vi "Update.vi"(8 "error in (no error)":errorcluster caption="entrée d'erreur (pas d'erreur)", 11 "Database Drivers en entrée":refnum<class "Database Drivers.lvclass">) -> (0 "error out":errorcluster caption="sortie d'erreur", 3 "Database Drivers en sortie":refnum<class "Database Drivers.lvclass">)   [LabVIEW 2020, in "Library Instrument & Equipement.lvlib" / "Library Database.lvlib" / "Database Drivers.lvclass"]
uses:
  Database Drivers.lvclass
  <vilib>/addons/database/Command.llb/Cmd Execute.vi
  <vilib>/addons/database/Recordset.llb/Rec Destroy - Command.vi
  <vilib>/addons/database/Command.llb/Cmd Delete.vi
  Database Drivers.lvclass/Database Drivers.ctl
  <vilib>/addons/database/NI_Database_API.lvlib
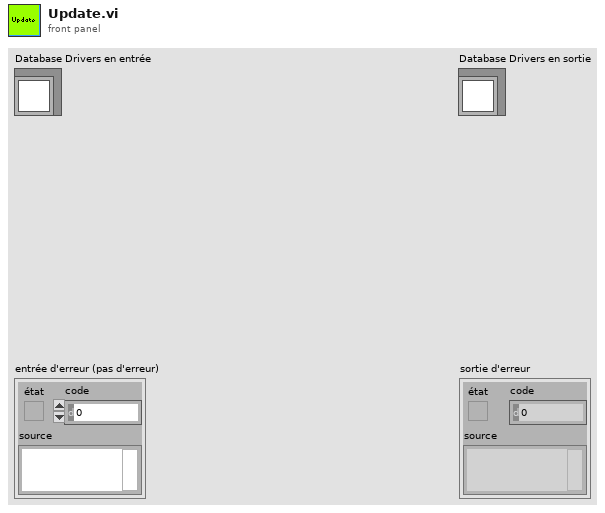
[diagram p1: front panel]
types:
  T1 = typedef "NI_Database_API.lvlib/Conn ObjectReference.ctl" = refnum<k1>
  T2 = typedef "NI_Database_API.lvlib/DB Tools Parameter Info.ctl" = cluster{"parameter name":string, "type":T3, "direction":T4, "value":variant}
  T3 = typedef "NI_Database_API.lvlib/DB Tools DataTypes.ctl" = enum16{"String", "Long (I32)", "Single (SGL)", "Double (DBL)", "Date/Time", "Binary"}
  T4 = typedef "NI_Database_API.lvlib/DB Tools Parameter Dir.ctl" = enum32{"Input", "Output", "Input/Output", "Return Value"}
  T5 = typedef "NI_Database_API.lvlib/Cmd ObjectReference.ctl" = refnum<k1>
  T6 = typedef "NI_Database_API.lvlib/Cmd-Rec Object Reference.ctl" = refnum<k1>
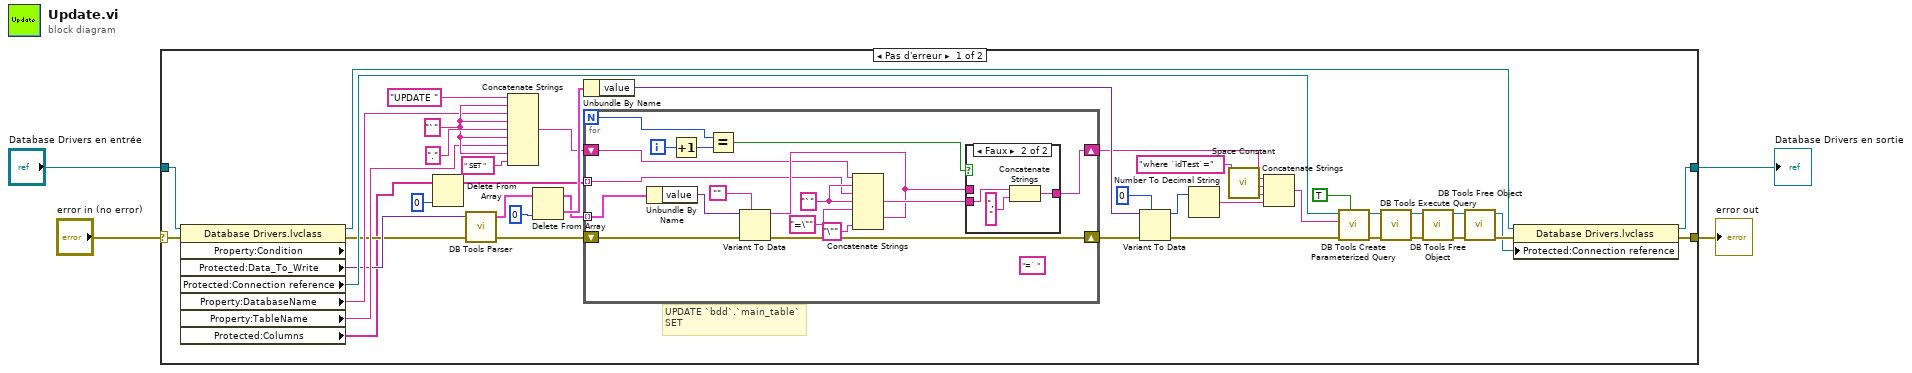
[diagram p0: block diagram]
diagram:
  n1 = case shown="Pas d'erreur" "error in (no error)" {
    selector: "error in (no error)" -> [w45 w69]
    tunnel: [w44 w69] -> w3
    tunnel: [w42 w68] -> w1
    tunnel: "Database Drivers en entrée" -> [w46 w68]
    frame No Error {
      w40 = "`" ("chaîne")
      # "UPDATE `bdd`.`main_table`\nSET"
      n2 = property class="Database Drivers.lvclass" props=["Property:Condition", "Protected:Data_To_Write", "Protected:Connection reference", "Property:DatabaseName", "Property:TableName", "Protected:Columns"](reference=w46, error in=w45) -> (reference out=w43:refnum<class "Database Drivers.lvclass">, error out=w16:errorcluster, "Protected:Data_To_Write"=w21:variant, "Protected:Connection reference"=w23:T1, "Property:DatabaseName"=w39:string, "Property:TableName"=w24:string, "Protected:Columns"=w7:string[])  [unwired: 1 out]
      n3 = Delete From Array(array=w7, index=0 ("indice")) -> (array with subset deleted=w5:string[])  [unwired: 1 in, 1 out]
      n4 = call <vilib>:"DB Tools Parser.vi"("error in (no error)"=w16, "variant"=w21) -> ("error out"=w17:errorcluster, "parameters"=w9:T2[])  [unwired: 2 in]
      n5 = Concatenate Strings("UPDATE " ("chaîne"), w40, w39, w40, "." ("chaîne"), w40, w24, w40, " SET " ("chaîne")) -> (w10:string)
      n6 = Delete From Array(array=w9, index=0 ("indice")) -> (deleted portion=w20:T2, array with subset deleted=w8:T2[])  [unwired: 1 in]
      n7 = Unbundle By Name(w20) -> ("value"=w19:variant)
      n8 = for {
        N -> [w52]
        shift-right: [w60] -> w18
        shift-left: w17 -> [w61]
        shift-right: [w57] -> w15
        shift-left: w10 -> [w56]
        tunnel: w5 -> [w53] mode=indexing
        tunnel: w8 -> [w48] mode=indexing
        i -> [w51]
        w54 = "`" ("chaîne")
        (unwired) "=` "
        n9 = Unbundle By Name(w48) -> ("value"=w63:variant)
        n10 = Increment(x=w51) -> (x+1=w49:i32)
        n11 = Equal?(x=w52, y=w49) -> (x = y?=w50:bool)
        n12 = Variant To Data(error in=w61, type="", Variant=w63) -> (data=w58:string, error out=w60:errorcluster)
        n13 = Concatenate Strings(w56, w54, w53, w54, "=\"", w58, "\"" ("chaîne")) -> (w59:string)
        n14 = case shown="Faux" w50 {
          tunnel: w59 -> [w64 w66]
          tunnel: [w64 w65] -> w57
          tunnel: w58 -> [_ _]
          frame True {
          }
          frame False {
            n15 = Concatenate Strings(w66, ", " ("Substring")) -> (w65:string)
          }
        }
      }
      n16 = Variant To Data(error in=w18, type=0, Variant=w19) -> (data=w35:i32, error out=w13:errorcluster)
      n17 = Number To Decimal String(number=w35) -> (decimal integer string=w34:string)  [unwired: 1 in]
      n18 = call <vilib>:"Space Constant.vi"() -> ("String"=w25:string)
      n19 = Concatenate Strings(w15, w25, "where `idTest`=" ("condition"), w34) -> (w14:string)
      n20 = call <vilib>:"DB Tools Create Parameterized Query.vi"("auto-detect parameters? (F)"=TRUE, "error in (no error)"=w13, "SQL query"=w14, "connection reference"=w23) -> ("error out"=w32:errorcluster, "command reference"=w31:T5)  [unwired: 3 in, 1 out]
      n21 = call-poly <vilib>:"DB Tools Execute Query.vi"("error in (no error)"=w32, "command reference"=w31) -> ("error out"=w29:errorcluster, "command-recordset reference"=w30:T6)  [unwired: 6 in]
      n22 = call-poly <vilib>:"DB Tools Free Object.vi"("error in (no error)"=w29, "command-recordset reference"=w30) -> ("error out"=w33:errorcluster, "command reference"=w28:T5)  [unwired: 8 in]
      n23 = call-poly <vilib>:"DB Tools Free Object.vi"("error in (no error)"=w33, "command reference"=w28) -> ("error out"=w27:errorcluster, "connection reference"=w26:T1)  [unwired: 8 in]
      n24 = property class="Database Drivers.lvclass"(reference=w43, error in=w27, "Protected:Connection reference"=w26) -> (reference out=w42:refnum<class "Database Drivers.lvclass">, error out=w44:errorcluster)
    }
    frame Error {
    }
  }
  "error out" <- w3
  "Database Drivers en sortie" <- w1
